vi "Init.vi"(11 "Online?":bool) -> (0 "Fehler out":T1, 1 "SPS-Event":refnum<user-event>, 2 "Version":string, 3 "Cluster out":T2={"Initialisierung"={"Online?"=FALSE, "Grundpfad"=path "", "Kamera Oben"="", "IP-Adresse Flüssiglinse"="", "Flüssiglinse"=refnum, "Kamera Unten"="", "IP-Adresse SPS"="", "SPS-Verbindung"={"TCP Connection Ref"=refnum, "IP address"="", "timeout ms"=5000, "Connected?"=FALSE, "PLC Type"=enum."S7 1200", "Rack S7 400"=0, "Slot S7 400"=0, "PDU Size"=0, "connection semaphore"=refnum}, "IP-Adresse Lichtgitter"="", "Lichtgitter"=refnum, "Skalierungsfaktor"=0.0, "Bilder Oben"=[], "Bild Unten"=refnum, "Bild Ausschnitt Unten"=refnum}, "Einstellungen"={"Gesamtablauf gestartet"=FALSE, "i. O. Bilder speichern"=FALSE, "Bildspeicherung Offline"=FALSE, "Ausgewähltes Offline-Datum"="", "Ausgewähltes Offline-Teil"="", "Speicherpfad Bilder"=path ""}, "Artikeldaten"={"Artikelnummer"="", "Fertigungsauftrag"="", "Muster ISO"=refnum, "Belichtungszeit Referenzmarken"=0.0, "Fokus Referenzmarken"=0.0, "Belichtungszeit ISO"=0.0, "Fokus ISO"=0.0, "Belichtungszeit Unten"=0.0, "Kontaktanzahl"=0, "Aktueller Kontakt"=0, "Kontaktposition"={"x"=0.0, "y"=0.0}, "ISO-Muster nicht vorhanden"=FALSE, "Winkel ISO"=0.0, "Mittelpunkt ISO"={"x"=0.0, "y"=0.0}}, "Werte Kamera Oben"={"Koordinatensystem"={"Punkt x-Achse"={"X"=0.0, "Y"=0.0}, "Ursprung"={"X"=0.0, "Y"=0.0}, "Punkt y-Achse"={"X"=0.0, "Y"=0.0}}, "Position Kontakt"={"x"=0.0, "y"=0.0}, "Durchmesser Loch"=0.0, "Winkel Kontakt"=0.0}, "Werte Kamera Unten"={"Prüfung Unten n. i. O."=FALSE}, "Werte Lichtgitter"={"Messwerte Referenzmarken"=[], "Mittelpunkt Referenzmarken"={"x"=0.0, "y"=0.0}, "Messwerte Kontakt"=[], "Offset"={"x"=0.0, "y"=0.0}}, "Rückmeldungen"={"Koordinaten ermittelt"=FALSE, "Vermessung Lichtgitter fertig"=FALSE, "Nachkontrolle Kamera Unten fertig"=FALSE}, "Fehler"={"Referenzen nicht gefunden"=FALSE, "Kontakt nicht gefunden"=FALSE, "Referenzen nicht in Lichtgitter"=FALSE, "Kontakt zu groß"=FALSE, "Kontakt zu klein"=FALSE}, "Statistik"={"Statistiken"=[]}, "Timer"={"Timer Start Position"=0, "Timer Start Lichtgitter"=0, "Timer Start Kamera Unten"=0}})   [LabVIEW 2024]
doc: "Verbindet alle Geräte und initialisiert Grundvariablen"
uses:
  Typdefinitionen/Cluster.ctl
  <vilib>/userDefined/High Color/IMAQdx.ctl
  <vilib>/DATA AHEAD/SP7/typedefs/S7 Connection.ctl
  <vilib>/DATA AHEAD/SP7/typedefs/PLC Type.ctl
  <vilib>/vision/Image Controls.llb/IMAQ Image.ctl
  Typdefinitionen/Koordinatensystem.ctl
  Typdefinitionen/Statistik.ctl
  Typdefinitionen/Cluster_Fehler_Initialisierung.ctl
  Typdefinitionen/Zustand.ctl
  <vilib>/Utility/config.llb/Read Key (String).vi
  Sonstige/Globale Variablen.vi
  <vilib>/Utility/config.llb/Read Key (Double).vi
  <vilib>/DATA AHEAD/SP7/SP7.lvlib
  <vilib>/vision/driver/NI_Vision_Acquisition_Software.lvlib
  <vilib>/Utility/config.llb/NI_LVConfig.lvlib
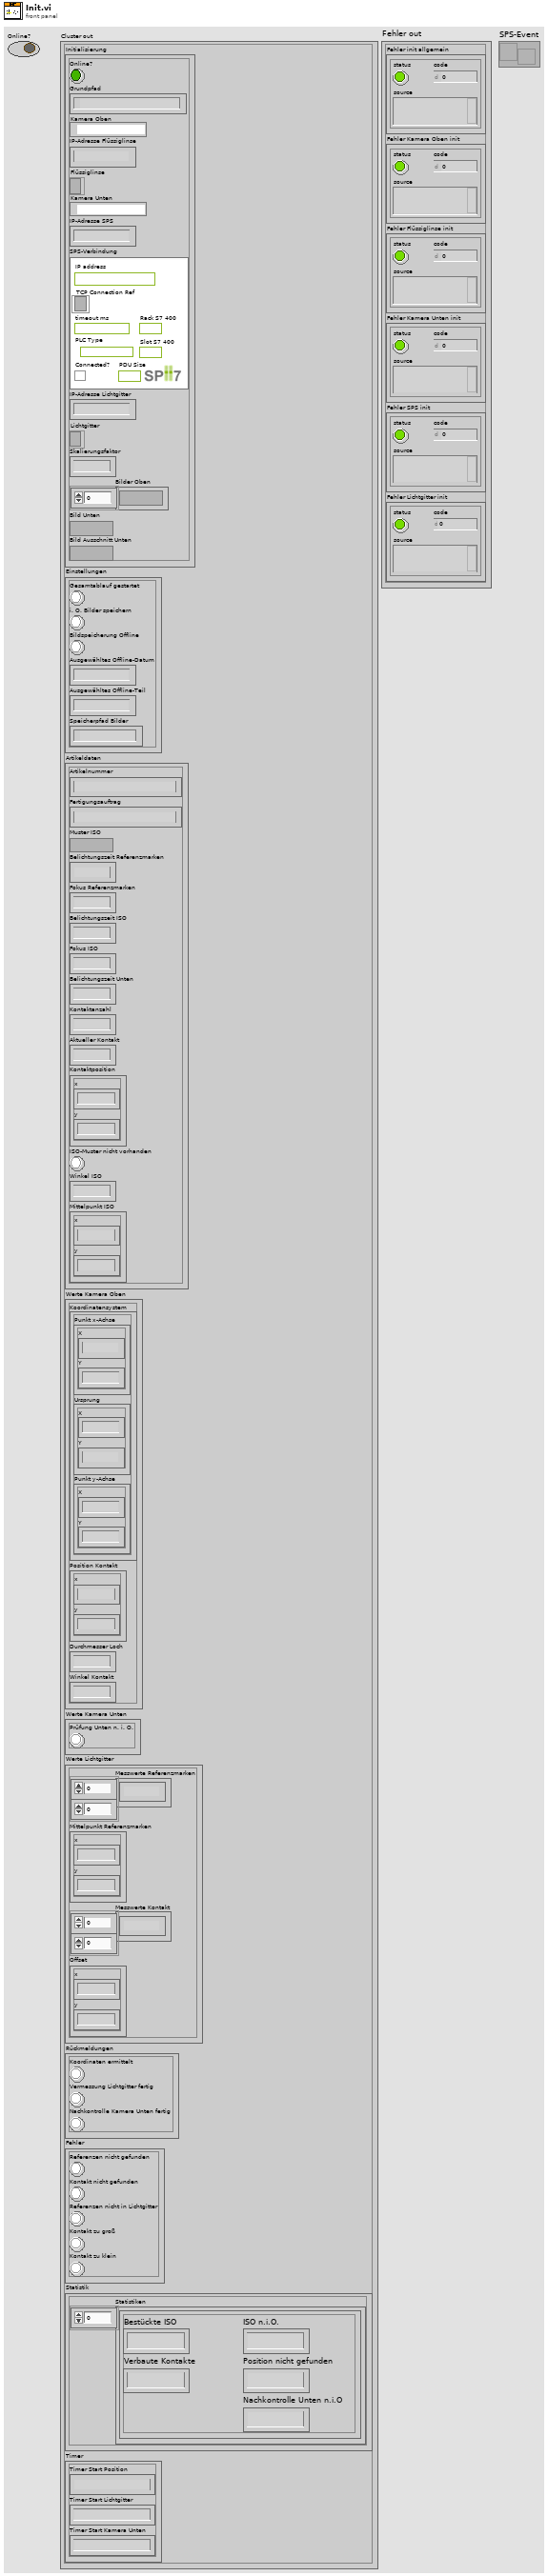
[diagram p1: front panel]
types:
  T1 = typedef "Cluster_Fehler_Initialisierung.ctl" = cluster{"Fehler init allgemein":errorcluster, "Fehler Kamera Oben init":errorcluster, "Fehler Flüssiglinse init":errorcluster, "Fehler Kamera Unten init":errorcluster, "Fehler SPS init":errorcluster, "Fehler Lichtgitter init":errorcluster}
  T2 = typedef "Cluster.ctl" = cluster{"Initialisierung":cluster{"Online?":bool, "Grundpfad":path, "Kamera Oben":T3, "IP-Adresse Flüssiglinse":string, "Flüssiglinse":refnum<k5>, "Kamera Unten":T3, "IP-Adresse SPS":string, "SPS-Verbindung":T4, "IP-Adresse Lichtgitter":string, "Lichtgitter":refnum<k5>, "Skalierungsfaktor":dbl, "Bilder Oben":T7[], "Bild Unten":T7, "Bild Ausschnitt Unten":T7}, "Einstellungen":cluster{"Gesamtablauf gestartet":bool, "i. O. Bilder speichern":bool, "Bildspeicherung Offline":bool, "Ausgewähltes Offline-Datum":string, "Ausgewähltes Offline-Teil":string, "Speicherpfad Bilder":path}, "Artikeldaten":cluster{"Artikelnummer":string, "Fertigungsauftrag":string, "Muster ISO":T7, "Belichtungszeit Referenzmarken":dbl, "Fokus Referenzmarken":dbl, "Belichtungszeit ISO":dbl, "Fokus ISO":dbl, "Belichtungszeit Unten":dbl, "Kontaktanzahl":u32, "Aktueller Kontakt":i16, "Kontaktposition":cluster{"x":sgl, "y":sgl}, "ISO-Muster nicht vorhanden":bool, "Winkel ISO":sgl, "Mittelpunkt ISO":cluster{"x":dbl, "y":dbl}}, "Werte Kamera Oben":cluster{"Koordinatensystem":T8, "Position Kontakt":cluster{"x":dbl, "y":dbl}, "Durchmesser Loch":dbl, "Winkel Kontakt":dbl}, "Werte Kamera Unten":cluster{"Prüfung Unten n. i. O.":bool}, "Werte Lichtgitter":cluster{"Messwerte Referenzmarken":dbl[][], "Mittelpunkt Referenzmarken":cluster{"x":dbl, "y":dbl}, "Messwerte Kontakt":dbl[][], "Offset":cluster{"x":dbl, "y":dbl}}, "Rückmeldungen":cluster{"Koordinaten ermittelt":bool, "Vermessung Lichtgitter fertig":bool, "Nachkontrolle Kamera Unten fertig":bool}, "Fehler":cluster{"Referenzen nicht gefunden":bool, "Kontakt nicht gefunden":bool, "Referenzen nicht in Lichtgitter":bool, "Kontakt zu groß":bool, "Kontakt zu klein":bool}, "Statistik":cluster{"Statistiken":T9[]}, "Timer":cluster{"Timer Start Position":u32, "Timer Start Lichtgitter":u32, "Timer Start Kamera Unten":u32}}
  T3 = typedef "IMAQdx.ctl" = refnum<k21>
  T4 = typedef "SP7.lvlib/S7 Connection.ctl" = cluster{"TCP Connection Ref":refnum<k5>, "IP address":string, "timeout ms":i32, "Connected?":bool, "PLC Type":T5, "Rack S7 400":u8, "Slot S7 400":u8, "PDU Size":u16, "connection semaphore":T6}
  T5 = typedef "SP7.lvlib/PLC Type.ctl" = enum16{"S7 200", "S7 300/400", "S7 1200", "S7 1500", "LOGO!8"}
  T6 = typedef "Semaphore RefNum" = refnum<k1>
  T7 = typedef "IMAQ Image.ctl" = refnum<image>
  T8 = typedef "Koordinatensystem.ctl" = cluster{"Punkt x-Achse":cluster{"X":sgl, "Y":sgl}, "Ursprung":cluster{"X":sgl, "Y":sgl}, "Punkt y-Achse":cluster{"X":sgl, "Y":sgl}}
  T9 = typedef "Statistik.ctl" = cluster{"Bestückte ISO":u32, "Verbaute Kontakte":u32, "ISO n.i.O.":u32, "Nachkontrolle Unten n.i.O":u32, "Position nicht gefunden":u32}
  T10 = typedef "Zustand.ctl" = enum16{"Warten auf Event", "Artikeldaten laden", "Init Prüfung Oben", "Bildaufnahme Oben", "Auswertung Oben", "Bilder Oben speichern", "Init Vermessung Lichtgitter", "Messwertaufnahme Lichtgitter", "Auswertung Lichtgitter", "Init Prüfung Unten", "Bildaufnahme Unten", "Auswertung Unten", "Bild Unten speichern", "Update Statistik", "Fehler quittieren"}
  T11 = typedef "NI_LVConfig.lvlib/Config Data RefNum.ctl" = refnum<k1>
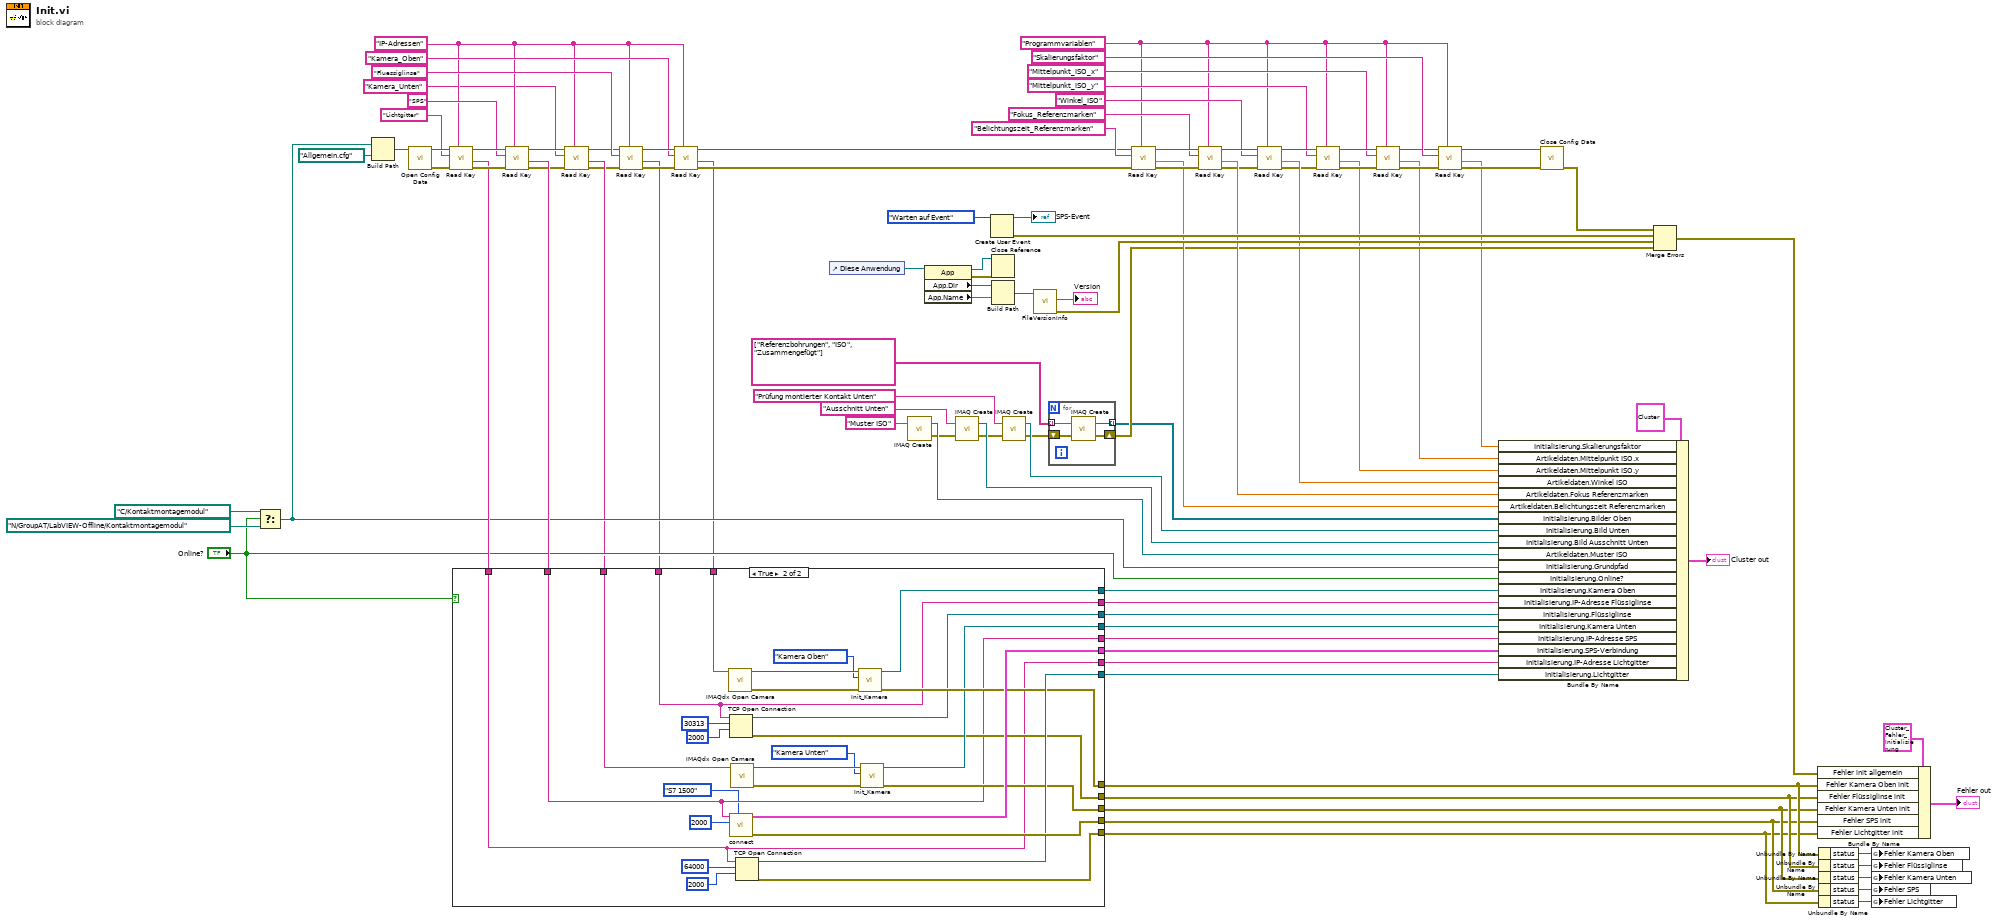
[diagram p0: block diagram]
diagram:
  w29 = "IP-Adressen" ("section")
  w1 = "Programmvariablen" ("section")
  n1 = Select(t=path "C:/Kontaktmontagemodul", s="Online?", f=path "N:/GroupAT/LabVIEW-Offline/Kontaktmontagemodul") -> (s? t:f=w41:path)
  n2 = Build Path(base path=w41, name or relative path=path "Allgemein.cfg") -> (appended path=w75:path)
  n3 = call <vilib>:"Open Config Data.vi"("configuration file path"=w75) -> ("error out"=w60:errorcluster, "refnum"=w61:T11)  [unwired: 8 in, 1 out]
  n4 = call-poly <vilib>:"Read Key.vi"("section"=w29, "error in (no error)"=w60, "key"="Lichtgitter", "refnum"=w61) -> ("error out"=w58:errorcluster, "value"=w53:string, "refnum out"=w59:T11)  [unwired: 4 in, 1 out]
  n5 = call-poly <vilib>:"Read Key.vi"("section"=w29, "error in (no error)"=w58, "key"="SPS", "refnum"=w59) -> ("error out"=w30:errorcluster, "value"=w54:string, "refnum out"=w34:T11)  [unwired: 4 in, 1 out]
  n6 = call-poly <vilib>:"Read Key.vi"("section"=w29, "error in (no error)"=w30, "key"="Kamera_Unten", "refnum"=w34) -> ("error out"=w31:errorcluster, "value"=w32:string, "refnum out"=w33:T11)  [unwired: 4 in, 1 out]
  n7 = call-poly <vilib>:"Read Key.vi"("section"=w29, "error in (no error)"=w31, "key"="Fluessiglinse", "refnum"=w33) -> ("error out"=w40:errorcluster, "value"=w27:string, "refnum out"=w39:T11)  [unwired: 4 in, 1 out]
  n8 = call-poly <vilib>:"Read Key.vi"("section"=w29, "error in (no error)"=w40, "key"="Kamera_Oben", "refnum"=w39) -> ("error out"=w37:errorcluster, "value"=w36:string, "refnum out"=w38:T11)  [unwired: 4 in, 1 out]
  n9 = case shown="True" "Online?" {
    tunnel: [_ w128] -> w44
    tunnel: [_ w120] -> w52
    tunnel: [_ w127] -> w43
    tunnel: [_ w115] -> w45
    tunnel: [_ w118] -> w93
    tunnel: [_ w114] -> w92
    tunnel: [_ w126] -> w91
    tunnel: [_ w125] -> w90
    tunnel: [_ w106] -> w82
    tunnel: [_ w105] -> w83
    tunnel: [_ w110] -> w81
    tunnel: [_ w107] -> w80
    tunnel: [_ w109] -> w46
    tunnel: w27 -> [_ w107]
    tunnel: w54 -> [_ w106]
    tunnel: w53 -> [_ w105]
    tunnel: w36 -> [_ w104]
    tunnel: w32 -> [_ w103]
    frame False {
    }
    frame True {
      n10 = call <vilib>:"IMAQdx Open Camera.vi"("Session In"=w104) -> ("error out"=w121:errorcluster, "Session Out"=w119:T3)  [unwired: 9 in]
      n11 = TCP Open Connection(address=w107, remote port or service name=u16 30313 ("Netzwerk-Port oder -Dienst"), timeout ms (60000)=2000) -> (connection ID=w110:refnum<k5>, error out=w109:errorcluster)  [unwired: 2 in]
      n12 = call <vilib>:"connect.vi"("PLC Type"=PLC_Type."S7 1500", "timeout [ms]"=2000, "IP address"=w106) -> ("error out"=w128:errorcluster, "S7 Connection out"=w126:T4)  [unwired: 7 in]
      n13 = call <vilib>:"IMAQdx Open Camera.vi"("Session In"=w103) -> ("error out"=w117:errorcluster, "Session Out"=w116:T3)  [unwired: 9 in]
      n14 = TCP Open Connection(address=w105, remote port or service name=u16 64000, timeout ms (60000)=2000) -> (connection ID=w125:refnum<k5>, error out=w127:errorcluster)  [unwired: 2 in]
      n15 = call "Init_Kamera.vi"("Fehler in"=w121, "Kamera"=enum16{"Kamera Oben", "Kamera Unten"}."Kamera Oben", "Kamera in"=w119) -> ("Fehler out"=w120:errorcluster, "Kamera out"=w118:T3)  [unwired: 7 in]
      n16 = call "Init_Kamera.vi"("Fehler in"=w117, "Kamera"=enum16{"Kamera Oben", "Kamera Unten"}."Kamera Unten", "Kamera in"=w116) -> ("Fehler out"=w115:errorcluster, "Kamera out"=w114:T3)  [unwired: 7 in]
    }
  }
  n17 = control-ref of="Diese Anwendung"() -> (w101:refnum<vi>)
  n18 = call "IMAQ Create"("Image Name"="Muster ISO") -> ("New Image"=w17:T7, "error out"=w16:errorcluster)  [unwired: 4 in]
  n19 = property class="App"(reference=w101) -> (reference out=w97:refnum<vi>, error out=w98:errorcluster, "App.Dir"=w99:path, "App.Name"=w100:string)  [unwired: 1 in]
  n20 = call "IMAQ Create"("Image Name"="Ausschnitt Unten", "error in (no error)"=w16) -> ("New Image"=w22:T7, "error out"=w15:errorcluster)  [unwired: 3 in]
  n21 = Create User Event(user event datatype=Zustand."Warten auf Event" ("Enum")) -> (user event=→"SPS-Event":refnum<user-event>, error out=w78:errorcluster)  [unwired: 1 in]
  n22 = Close Reference(reference=w97, error in (no error)=w98) -> ()  [unwired: 1 out]
  n23 = Build Path(base path=w99, name or relative path=w100) -> (appended path=w96:path)
  n24 = call "IMAQ Create"("Image Name"="Prüfung montierter Kontakt Unten", "error in (no error)"=w15) -> ("New Image"=w85:T7, "error out"=w14:errorcluster)  [unwired: 3 in]
  n25 = call "FileVersionInfo.vi"("Application Path in"=w96) -> ("error out"=w87:errorcluster, "File Version Info"=→"Version":string)  [unwired: 7 in, 2 out]
  n26 = for {
    shift-right: [w132] -> w66
    shift-left: w14 -> [w131]
    tunnel: string[] ["Referenzbohrungen", "ISO", "Zusammengefügt"] -> [w130] mode=indexing
    tunnel: [w129] -> w65 mode=indexing
    n27 = call "IMAQ Create"("Image Name"=w130, "error in (no error)"=w131) -> ("New Image"=w129:T7, "error out"=w132:errorcluster)  [unwired: 3 in]
  }
  n28 = call-poly <vilib>:"Read Key.vi"("section"=w1, "error in (no error)"=w37, "key"="Belichtungszeit_Referenzmarken", "refnum"=w38) -> ("error out"=w71:errorcluster, "value"=w69:dbl, "refnum out"=w72:T11)  [unwired: 4 in, 1 out]
  n29 = call-poly <vilib>:"Read Key.vi"("section"=w1, "error in (no error)"=w71, "key"="Fokus_Referenzmarken", "refnum"=w72) -> ("error out"=w20:errorcluster, "value"=w68:dbl, "refnum out"=w21:T11)  [unwired: 4 in, 1 out]
  n30 = call-poly <vilib>:"Read Key.vi"("section"=w1, "error in (no error)"=w20, "key"="Winkel_ISO", "refnum"=w21) -> ("error out"=w9:errorcluster, "value"=w18:dbl, "refnum out"=w8:T11)  [unwired: 4 in, 1 out]
  n31 = call-poly <vilib>:"Read Key.vi"("section"=w1, "error in (no error)"=w9, "key"="Mittelpunkt_ISO_y", "refnum"=w8) -> ("error out"=w10:errorcluster, "value"=w5:dbl, "refnum out"=w11:T11)  [unwired: 4 in, 1 out]
  n32 = call-poly <vilib>:"Read Key.vi"("section"=w1, "error in (no error)"=w10, "key"="Mittelpunkt_ISO_x", "refnum"=w11) -> ("error out"=w7:errorcluster, "value"=w4:dbl, "refnum out"=w6:T11)  [unwired: 4 in, 1 out]
  n33 = call-poly <vilib>:"Read Key.vi"("section"=w1, "error in (no error)"=w7, "key"="Skalierungsfaktor" ("section"), "refnum"=w6) -> ("error out"=w25:errorcluster, "value"=w13:dbl, "refnum out"=w26:T11)  [unwired: 4 in, 1 out]
  n34 = Bundle By Name(cluster=T2 {"Initialisierung"={"Online?"=FALSE, "Grundpfad"=path "N:/GroupAT/LabVIEW-Offline/Kontaktmontagemodul", "Kamera Oben"="", "IP-Adresse Flüssiglinse"="", "Flüssiglinse"=refnum, "Kamera Unten"="", "IP-Adresse SPS"="", "SPS-Verbindung"={"TCP Connection Ref"=refnum, "IP address"="", "timeout ms"=0, "Connected?"=FALSE, "PLC Type"=enum."S7 200", "Rack S7 400"=0, "Slot S7 400"=0, "PDU Size"=0, "connection semaphore"=refnum}, "IP-Adresse Lichtgitter"="", "Lichtgitter"=refnum, "Skalierungsfaktor"=0.0, "Bilder Oben"=["remote image 00000000108EE02C", "remote image 00000000108EE12C", "remote image 00000000108EE82C"], "Bild Unten"="remote image 00000000108EE1AC", "Bild Ausschnitt Unten"=refnum}, "Einstellungen"={"Gesamtablauf gestartet"=FALSE, "i. O. Bilder speichern"=FALSE, "Bildspeicherung Offline"=FALSE, "Ausgewähltes Offline-Datum"="12.07.24", "Ausgewähltes Offline-Teil"="0", "Speicherpfad Bilder"=path "N:/GroupAT/LabVIEW-Offline/Kontaktmontagemodul/Artikelnummern/Test/Bilder/23.08.24/2"}, "Artikeldaten"={"Artikelnummer"="", "Fertigungsauftrag"="", "Muster ISO"=refnum, "Belichtungszeit Referenzmarken"=1000.0, "Fokus Referenzmarken"=-2.0, "Belichtungszeit ISO"=0.0, "Fokus ISO"=0.0, "Belichtungszeit Unten"=0.0, "Kontaktanzahl"=0, "Aktueller Kontakt"=1, "Kontaktposition"={"x"=0.0, "y"=0.0}, "ISO-Muster nicht vorhanden"=FALSE, "Winkel ISO"=0.0, "Mittelpunkt ISO"={"x"=0.0, "y"=0.0}}, "Werte Kamera Oben"={"Koordinatensystem"={"Punkt x-Achse"={"X"=0.0, "Y"=0.0}, "Ursprung"={"X"=0.0, "Y"=0.0}, "Punkt y-Achse"={"X"=0.0, "Y"=0.0}}, "Position Kontakt"={"x"=0.0, "y"=0.0}, "Durchmesser Loch"=0.0, "Winkel Kontakt"=0.0}, "Werte Kamera Unten"={"Prüfung Unten n. i. O."=FALSE}, "Werte Lichtgitter"={"Messwerte Referenzmarken"=[], "Mittelpunkt Referenzmarken"={"x"=0.0, "y"=0.0}, "Messwerte Kontakt"=[], "Offset"={"x"=0.0, "y"=0.0}}, "Rückmeldungen"={"Koordinaten ermittelt"=FALSE, "Vermessung Lichtgitter fertig"=FALSE, "Nachkontrolle Kamera Unten fertig"=FALSE}, "Fehler"={"Referenzen nicht gefunden"=FALSE, "Kontakt nicht gefunden"=FALSE, "Referenzen nicht in Lichtgitter"=FALSE, "Kontakt zu groß"=FALSE, "Kontakt zu klein"=FALSE}, "Statistik"={"Statistiken"=[]}, "Timer"={"Timer Start Position"=0, "Timer Start Lichtgitter"=0, "Timer Start Kamera Unten"=0}} ("Cluster out"), "Initialisierung.Skalierungsfaktor"=w13, "Artikeldaten.Mittelpunkt ISO.x"=w4, "Artikeldaten.Mittelpunkt ISO.y"=w5, "Artikeldaten.Winkel ISO"=w18, "Artikeldaten.Fokus Referenzmarken"=w68, "Artikeldaten.Belichtungszeit Referenzmarken"=w69, "Initialisierung.Bilder Oben"=w65, "Initialisierung.Bild Unten"=w85, "Initialisierung.Bild Ausschnitt Unten"=w22, "Artikeldaten.Muster ISO"=w17, "Initialisierung.Grundpfad"=w41, "Initialisierung.Online?"="Online?", "Initialisierung.Kamera Oben"=w93, "Initialisierung.IP-Adresse Flüssiglinse"=w80, "Initialisierung.Flüssiglinse"=w81, "Initialisierung.Kamera Unten"=w92, "Initialisierung.IP-Adresse SPS"=w82, "Initialisierung.SPS-Verbindung"=w91, "Initialisierung.IP-Adresse Lichtgitter"=w83, "Initialisierung.Lichtgitter"=w90) -> (→"Cluster out":T2)
  n35 = call <vilib>:"Close Config Data.vi"("error in (no error)"=w25, "refnum"=w26) -> ("error out"=w74:errorcluster)  [unwired: 8 in, 1 out]
  n36 = Merge Errors(w74, w78, w87, w66) -> (w64:errorcluster)
  n37 = Bundle By Name(cluster=T1 {"Fehler init allgemein"={"status"=FALSE, "code"=0, "source"=""}, "Fehler Kamera Oben init"={"status"=FALSE, "code"=0, "source"=""}, "Fehler Flüssiglinse init"={"status"=FALSE, "code"=0, "source"=""}, "Fehler Kamera Unten init"={"status"=FALSE, "code"=0, "source"=""}, "Fehler SPS init"={"status"=FALSE, "code"=0, "source"=""}, "Fehler Lichtgitter init"={"status"=FALSE, "code"=0, "source"=""}} ("Cluster"), "Fehler init allgemein"=w64, "Fehler Kamera Oben init"=w52, "Fehler Flüssiglinse init"=w46, "Fehler Kamera Unten init"=w45, "Fehler SPS init"=w44, "Fehler Lichtgitter init"=w43) -> (→"Fehler out":T1)
  n38 = Unbundle By Name(w52) -> ("status"=w51:bool)
  n39 = Unbundle By Name(w46) -> ("status"=w50:bool)
  n40 = Unbundle By Name(w45) -> ("status"=w49:bool)
  n41 = Unbundle By Name(w44) -> ("status"=w48:bool)
  n42 = Unbundle By Name(w43) -> ("status"=w47:bool)
  n43 = global write "Globale Variablen.vi" "Fehler Kamera Oben"(w51) -> ()
  n44 = global write "Globale Variablen.vi" "Fehler Flüssiglinse"(w50) -> ()
  n45 = global write "Globale Variablen.vi" "Fehler Kamera Unten"(w49) -> ()
  n46 = global write "Globale Variablen.vi" "Fehler SPS"(w48) -> ()
  n47 = global write "Globale Variablen.vi" "Fehler Lichtgitter"(w47) -> ()
